vi "Simple Dual Mode Thermometer Facade.vi"(0 "Data In":T4, 2 "Display State In":T2, 3 "Container State":T3) -> (6 "Data Out":T4, 7 "Display State Out":T2, 8 "Action":T1)   [LabVIEW 2020, in "Simple Dual Mode Thermometer XControl.xctl"]
doc: "This VI demonstrates the use of an XControl's Facade VI in implementing a Simple Dual Mode Thermometer. The front panel defines the appearance of the XControl. The block diagram defines the behavior of the XControl."
uses:
  Simple Dual Mode Thermometer XControl.xctl
  Simple Dual Mode Thermometer Data.ctl
  <vilib>/_xctls/Container State.ctl
  Simple Dual Mode Thermometer State.ctl
  <vilib>/_xctls/Action.ctl
  <vilib>/_xctls/XControlSupport.lvlib
panel:
  in  "format string":string="The temperature is %f degrees C or %f degrees F."
  in  "Item Name":string="Display Temperature..."
  in  "Action Name":string="Mode Change"
  in  "Fahrenheit":bool
  in  "Slide":dbl(slide) scale=0.0..100.0
  in  "Thermometer":dbl(slide) scale=0.0..100.0
  # "1. Drop the controls that make up the appearance\nof the XControl here.\n\n2. Resize the window to fit the controls\n\n3. If the XControl is of fixed size,  make the \n window not resizable from VI Properties->Window Appearance.\n\n4. If you want the controls to automatically size when the XControl sizes, check  \"Scale all objects on front panel when window resizes\" in File->VI Properties->Window Size page."
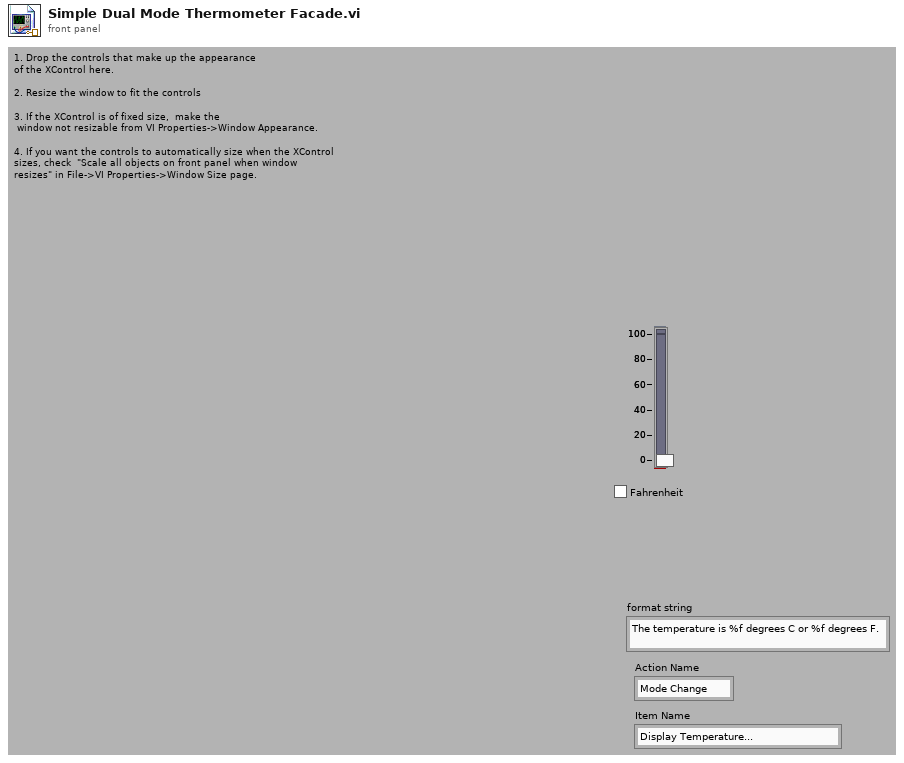
[diagram p1: front panel]
types:
  T1 = typedef "XControlSupport.lvlib/Action.ctl" = cluster{"Data Changed?":bool, "State Changed?":bool, "Action Name":string}
  T2 = typedef "Simple Dual Mode Thermometer XControl.xctl/Simple Dual Mode Thermometer State.ctl" = cluster{"Fahrenheit":bool}
  T3 = typedef "XControlSupport.lvlib/Container State.ctl" = cluster{"Indicator?":bool, "Run Mode?":bool, " Refnum":refnum<vi>}
  T4 = typedef "Simple Dual Mode Thermometer XControl.xctl/Simple Dual Mode Thermometer Data.ctl" = dbl
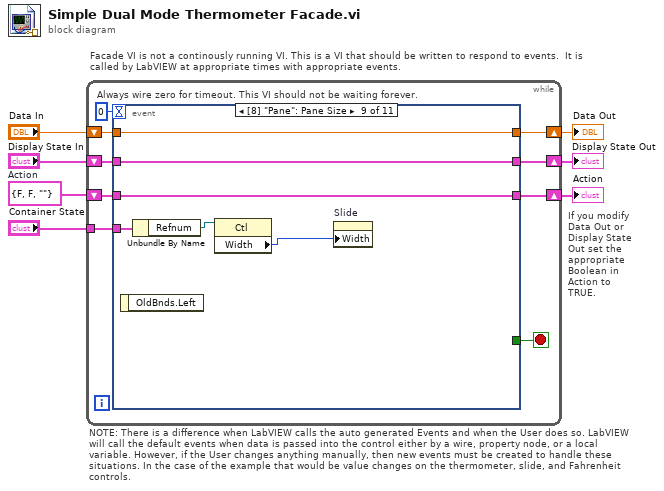
[diagram p0: block diagram]
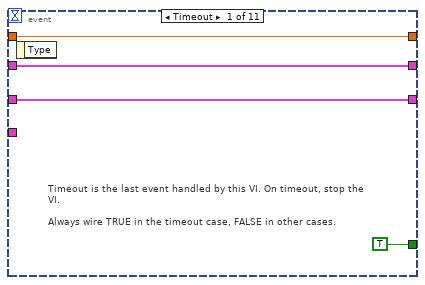
[diagram p2: hidden frame]
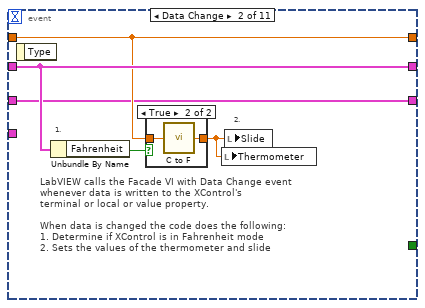
[diagram p3: hidden frame]
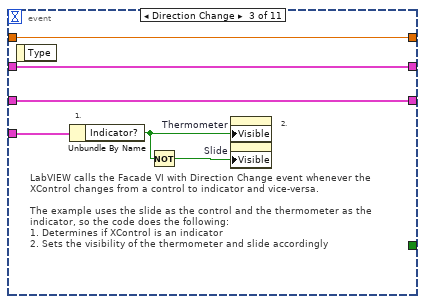
[diagram p5: hidden frame]
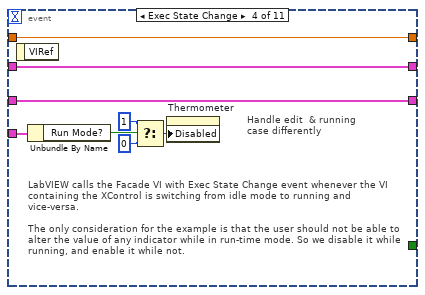
[diagram p6: hidden frame]
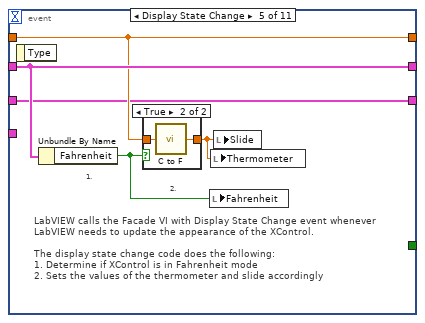
[diagram p7: hidden frame]
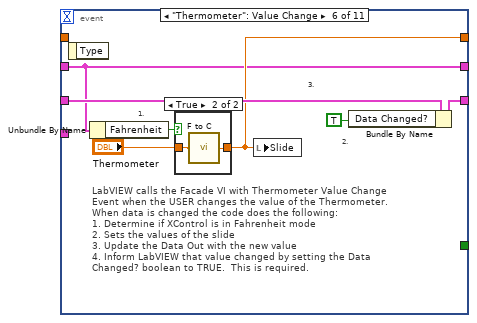
[diagram p9: hidden frame]
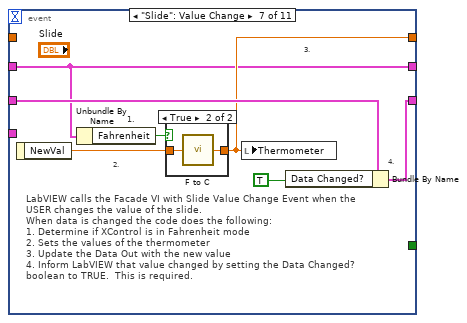
[diagram p11: hidden frame]
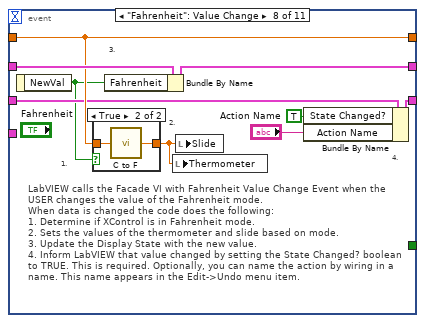
[diagram p13: hidden frame]
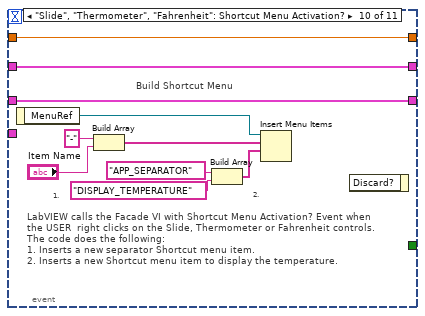
[diagram p15: hidden frame]
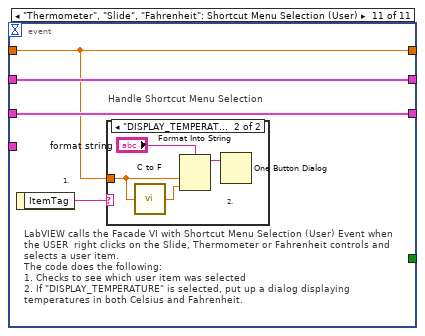
[diagram p16: hidden frame]
diagram:
  w1 = T1 {"Data Changed?"=FALSE, "State Changed?"=FALSE, "Action Name"=""}  # Action
  # "Facade VI is not a continously running VI. This is a VI that should be written to respond to events.  It is called by LabVIEW at appropriate times with appropriate events."
  # "NOTE: There is a difference when LabVIEW calls the auto generated Events and when the User does so. LabVIEW will call the default events when data is passed into the control either by a wire, property node, or a local variable. However, if the User changes anything manually, then new events must be created to handle these situations. In the case of the example that would be value changes on the thermometer, slide, and Fahrenheit controls."
  # "If you modify Data Out or Display State Out set the appropriate Boolean in Action to TRUE."
  n1 = while {
    shift-right: [w15] -> w4
    shift-left: "Display State In" -> [w16]
    tunnel: "Container State" -> [w12]
    shift-right: [w10] -> w7
    shift-left: "Data In" -> [w11]
    shift-right: [w8] -> w2
    shift-left: w1 -> [w9]
    stop <- w14 stop-if-true
    # "Always wire zero for timeout. This VI should not be waiting forever."
    n2 = event shown="[8] \"Pane\": Pane Size" {
      selector: _ -> [_ _ _ _ _ _ _ _ _ _ _]
      dyn-events: _ -> [_ _ _ _ _ _ _ _ _ _ _]
      timeout: 0 -> [_ _ _ _ _ _ _ _ _ _ _]
      tunnel: w16 -> [w18 w25 w33 w41 w47 w53 w62 w79 w87 w96 w101]
      tunnel: [w18 w25 w33 w41 w47 w53 w62 w78 w87 w96 w101] -> w15
      tunnel: [TRUE _ _ _ _ _ _ _ _ _ _] -> w14
      tunnel: w12 -> [_ _ w34 w42 _ _ _ _ w85 _ _]
      tunnel: w11 -> [w17 w23 w32 w40 w46 _ _ w77 w88 w97 w99]
      tunnel: [w17 w23 w32 w40 w46 w54 w63 w77 w88 w97 w99] -> w10
      tunnel: [w19 w21 w29 w39 w44 w55 w64 w73 w86 w98 w102] -> w8
      tunnel: w9 -> [w19 w21 w29 w39 w44 w56 w65 w76 w86 w98 w102]
      event Timeout {
        # "Timeout is the last event handled by this VI. On timeout, stop the VI.\n\nAlways wire TRUE in the timeout case, FALSE in other cases."
        n3 = event-data() -> ()  [unwired: 1 in, 1 out]
      }
      event Data Change {
        # "2."
        # "1."
        # "LabVIEW calls the Facade VI with Data Change event whenever data is written to the XControl's\nterminal or local or value property.\n \nWhen data is changed the code does the following:\n1. Determine if XControl is in Fahrenheit mode\n2. Sets the values of the thermometer and slide"
        n4 = event-data() -> ()  [unwired: 1 in, 1 out]
        n5 = Unbundle By Name(w25) -> ("Fahrenheit"=w24:bool)
        n6 = case shown="True" w24 {
          tunnel: w23 -> [w26 w28]
          tunnel: [w26 w27] -> w22
          frame False {
          }
          frame True {
            n7 = call "C to F.vi"("Celsius"=w28) -> ("Fahrenheit"=w27:dbl)
          }
        }
        n8 = local write "Thermometer"(w22) -> ()
        n9 = local write "Slide"(w22) -> ()
      }
      event Direction Change {
        # "2."
        # "1."
        # "LabVIEW calls the Facade VI with Direction Change event whenever the XControl changes from a control to indicator and vice-versa.\n\nThe example uses the slide as the control and the thermometer as the indicator, so the code does the following:\n1. Determines if XControl is an indicator\n2. Sets the visibility of the thermometer and slide accordingly"
        n10 = event-data() -> ()  [unwired: 1 in, 1 out]
        n11 = Unbundle By Name(w34) -> ("Indicator?"=w30:bool)
        n12 = Not(x=w30) -> (.not. x?=w31:bool)
        n13 = property on="Thermometer" class="Slide (strict)"("Visible"=w30) -> ()  [unwired: 2 in, 2 out]
        n14 = property on="Slide" class="Slide (strict)"("Visible"=w31) -> ()  [unwired: 2 in, 2 out]
      }
      event Exec State Change {
        # "LabVIEW calls the Facade VI with Exec State Change event whenever the VI containing the XControl is switching from idle mode to running and vice-versa.\n\nThe only consideration for the example is that the user should not be able to alter the value of any indicator while in run-time mode. So we disable it while running, and enable it while not."
        # "Handle edit  & running\ncase differently"
        n15 = event-data() -> ()  [unwired: 1 in, 1 out]
        n16 = Unbundle By Name(w42) -> ("Run Mode?"=w38:bool)
        n17 = Select(t=u8 1 ("Disabled"), s=w38, f=u8 0 ("Disabled")) -> (s? t:f=w35:u8)
        n18 = property on="Thermometer" class="Slide (strict)"("Disabled"=w35) -> ()  [unwired: 2 in, 2 out]
      }
      event Display State Change {
        # "2."
        # "1."
        # "LabVIEW calls the Facade VI with Display State Change event whenever LabVIEW needs to update the appearance of the XControl.\n\nThe display state change code does the following:\n1. Determine if XControl is in Fahrenheit mode\n2. Sets the values of the thermometer and slide accordingly"
        n19 = event-data() -> ()  [unwired: 1 in, 1 out]
        n20 = Unbundle By Name(w47) -> ("Fahrenheit"=w43:bool)
        n21 = case shown="True" w43 {
          tunnel: w46 -> [w48 w50]
          tunnel: [w48 w49] -> w45
          frame False {
          }
          frame True {
            n22 = call "C to F.vi"("Celsius"=w50) -> ("Fahrenheit"=w49:dbl)
          }
        }
        n23 = local write "Fahrenheit"(w43) -> ()
        n24 = local write "Thermometer"(w45) -> ()
        n25 = local write "Slide"(w45) -> ()
      }
      event "Thermometer": Value Change {
        # "LabVIEW calls the Facade VI with Thermometer Value Change Event when the USER changes the value of the Thermometer.\nWhen data is changed the code does the following:\n1. Determine if XControl is in Fahrenheit mode\n2. Sets the values of the slide\n3. Update the Data Out with the new value\n4. Inform LabVIEW that value changed by setting the Data Changed? boolean to TRUE.  This is required."
        # "3."
        # "2."
        # "1."
        n26 = event-data() -> ()  [unwired: 1 in, 1 out]
        n27 = Unbundle By Name(w53) -> ("Fahrenheit"=w52:bool)
        n28 = case shown="True" w52 {
          tunnel: "Thermometer" -> [w58 w59]
          tunnel: [w58 w60] -> w54
          frame False {
          }
          frame True {
            n29 = call "F to C.vi"("Fahrenheit"=w59) -> ("Celsius"=w60:dbl)
          }
        }
        n30 = local write "Slide"(w54) -> ()
        n31 = Bundle By Name(cluster=w56, "Data Changed?"=TRUE ("State Changed?")) -> (w55:T1)
      }
      event "Slide": Value Change {
        # "4."
        # "3."
        # "2."
        # "1."
        # "LabVIEW calls the Facade VI with Slide Value Change Event when the USER changes the value of the slide.\nWhen data is changed the code does the following:\n1. Determine if XControl is in Fahrenheit mode\n2. Sets the values of the thermometer\n3. Update the Data Out with the new value\n4. Inform LabVIEW that value changed by setting the Data Changed? boolean to TRUE.  This is required."
        n32 = event-data() -> ("NewVal"=w67:dbl)  [unwired: 1 in]
        n33 = Unbundle By Name(w62) -> ("Fahrenheit"=w61:bool)
        n34 = case shown="True" w61 {
          tunnel: w67 -> [w68 w70]
          tunnel: [w68 w69] -> w63
          frame False {
          }
          frame True {
            n35 = call "F to C.vi"("Fahrenheit"=w70) -> ("Celsius"=w69:dbl)
          }
        }
        n36 = local write "Thermometer"(w63) -> ()
        n37 = Bundle By Name(cluster=w65, "Data Changed?"=TRUE ("State Changed?")) -> (w64:T1)
      }
      event "Fahrenheit": Value Change {
        # "4."
        # "2."
        # "1."
        # "3."
        # "LabVIEW calls the Facade VI with Fahrenheit Value Change Event when the USER changes the value of the Fahrenheit mode.\nWhen data is changed the code does the following:\n1. Determine if XControl is in Fahrenheit mode.\n2. Sets the values of the thermometer and slide based on mode.\n3. Update the Display State with the new value.\n4. Inform LabVIEW that value changed by setting the State Changed? boolean to TRUE. This is required. Optionally, you can name the action by wiring in a name. This name appears in the Edit->Undo menu item."
        n38 = event-data() -> ("NewVal"=w72:bool)  [unwired: 1 in]
        n39 = case shown="True" w72 {
          tunnel: w77 -> [w80 w82]
          tunnel: [w80 w81] -> w71
          frame False {
          }
          frame True {
            n40 = call "C to F.vi"("Celsius"=w82) -> ("Fahrenheit"=w81:dbl)
          }
        }
        n41 = Bundle By Name(cluster=w79, "Fahrenheit"=w72) -> (w78:T2)
        n42 = local write "Thermometer"(w71) -> ()
        n43 = local write "Slide"(w71) -> ()
        n44 = Bundle By Name(cluster=w76, "State Changed?"=TRUE, "Action Name"="Action Name") -> (w73:T1)
      }
      event Pane Size {
        n45 = event-data() -> ()  [unwired: 1 in, 1 out]
        n46 = Unbundle By Name(w85) -> ("Refnum"=w84:refnum<vi>)
        n47 = property class="Ctl"(reference=w84) -> ("Width"=w83:u32)  [unwired: 1 in, 2 out]
        n48 = property on="Slide" class="Slide (strict)"("Width"=w83) -> ()  [unwired: 2 in, 2 out]
      }
      event "Slide", "Thermometer", "Fahrenheit": Shortcut Menu Activation? {
        # "Build Shortcut Menu"
        # "2."
        # "1."
        # "LabVIEW calls the Facade VI with Shortcut Menu Activation? Event when the USER  right clicks on the Slide, Thermometer or Fahrenheit controls.\nThe code does the following:\n1. Inserts a new separator Shortcut menu item.\n2. Inserts a new Shortcut menu item to display the temperature."
        n49 = event-data() -> ("MenuRef"=w92:refnum<k9>)  [unwired: 1 in]
        n50 = Build Array("-", "Item Name") -> (w93:string[])
        n51 = Build Array("APP_SEPARATOR", "DISPLAY_TEMPERATURE" ("element")) -> (w91:string[])
        n52 = Insert Menu Items(7:w91, 8:w93, 9:w92) -> ()  [unwired: 3 in, 3 out]
        n53 = event-data() -> ()  [unwired: 2 in, 1 out]
      }
      event "Thermometer", "Slide", "Fahrenheit": Shortcut Menu Selection (User) {
        # "Handle Shortcut Menu Selection"
        # "1."
        # "LabVIEW calls the Facade VI with Shortcut Menu Selection (User) Event when the USER  right clicks on the Slide, Thermometer or Fahrenheit controls and selects a user item.\nThe code does the following:\n1. Checks to see which user item was selected\n2. If \"DISPLAY_TEMPERATURE\" is selected, put up a dialog displaying temperatures in both Celsius and Fahrenheit."
        n54 = event-data() -> ("ItemTag"=w100:string)  [unwired: 1 in]
        n55 = case shown="\"DISPLAY_TEMPERATURE\"" w100 {
          tunnel: w99 -> [_ w103]
          frame Default {
          }
          frame "DISPLAY_TEMPERATURE" {
            # "2."
            n56 = call "C to F.vi"("Celsius"=w103) -> ("Fahrenheit"=w104:dbl)
            n57 = Format Into String(format string="format string", w103, w104) -> (resulting string=w105:string)  [unwired: 2 in, 1 out]
            n58 = One Button Dialog(message=w105) -> ()  [unwired: 1 in, 1 out]
          }
        }
      }
    }
  }
  "Display State Out" <- w4
  "Data Out" <- w7
  "Action" <- w2
